vi "LED Matrix Display TB.vi"() -> ()   [LabVIEW 2013]
panel:
  out "error out":errorcluster
  in  "Brightness":u8=50 max=100 step=1
  in  "Factor":dbl=1.0
  out "LED Matrix":picture
  in  "path to BMP file on myRio local filesystem":path=path "/home/admin/images/test.bmp"
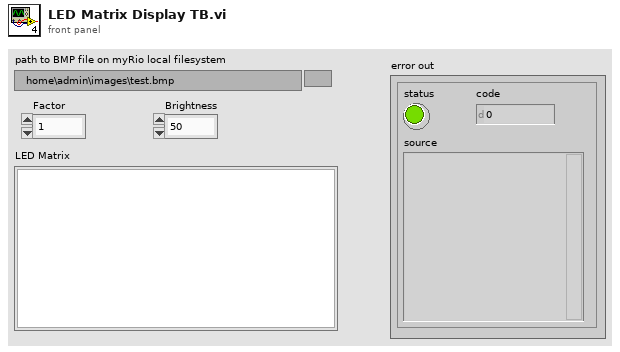
[diagram p1: front panel]
types:
  T1 = typedef "imagedata.ctl" = cluster{"image type":i32, "image depth":i32, "image":u8[], "mask":u8[], "colors":u32[], "Rectangle":cluster{"left":i16, "top":i16, "right":i16, "bottom":i16}}
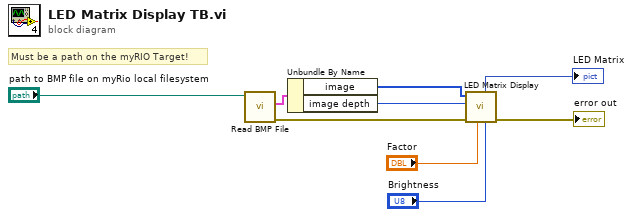
[diagram p0: block diagram]
diagram:
  # "Must be a path on the myRIO Target!"
  n1 = call <vilib>:"Read BMP File.vi"("path to BMP file"="path to BMP file on myRio local filesystem") -> ("error out"=w7:errorcluster, "image data"=w8:T1)  [unwired: 8 in, 1 out]
  n2 = Unbundle By Name(w8) -> ("image"=w6:u8[], "image depth"=w5:i32)
  n3 = call "LED Matrix Display.vi"("Brightness"="Brightness", "Factor"="Factor", "error in"=w7, "image depth"=w5, "image"=w6) -> ("error out"=→"error out":errorcluster, "LED Matrix"=→"LED Matrix":picture)  [unwired: 5 in]
